vi "Draw Line.vi"(6 "Colour":u32(colorbox), 9 "Point 2":T1, 10 "Point 1":T1, 11 "Pixels":refnum<data-value>) -> (3 "Pixels (dup)":refnum<data-value>)   [LabVIEW 2020, in "Raster.lvlib"]
uses:
  Raster.lvlib
  Point 2D.ctl
  <vilib>/Utility/High Resolution Relative Seconds.vi
  Utility/Utility.lvlib
panel:
  out "Processing Time [s]":dbl format="%.1p"
  out "Iteration":i32
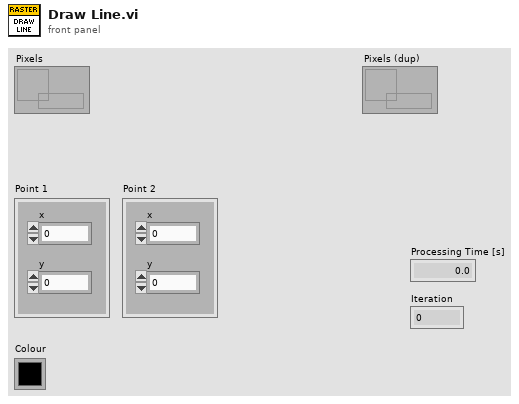
[diagram p1: front panel]
types:
  T1 = typedef "Raster.lvlib/Point 2D.ctl" = cluster{"x":i32, "y":i32}
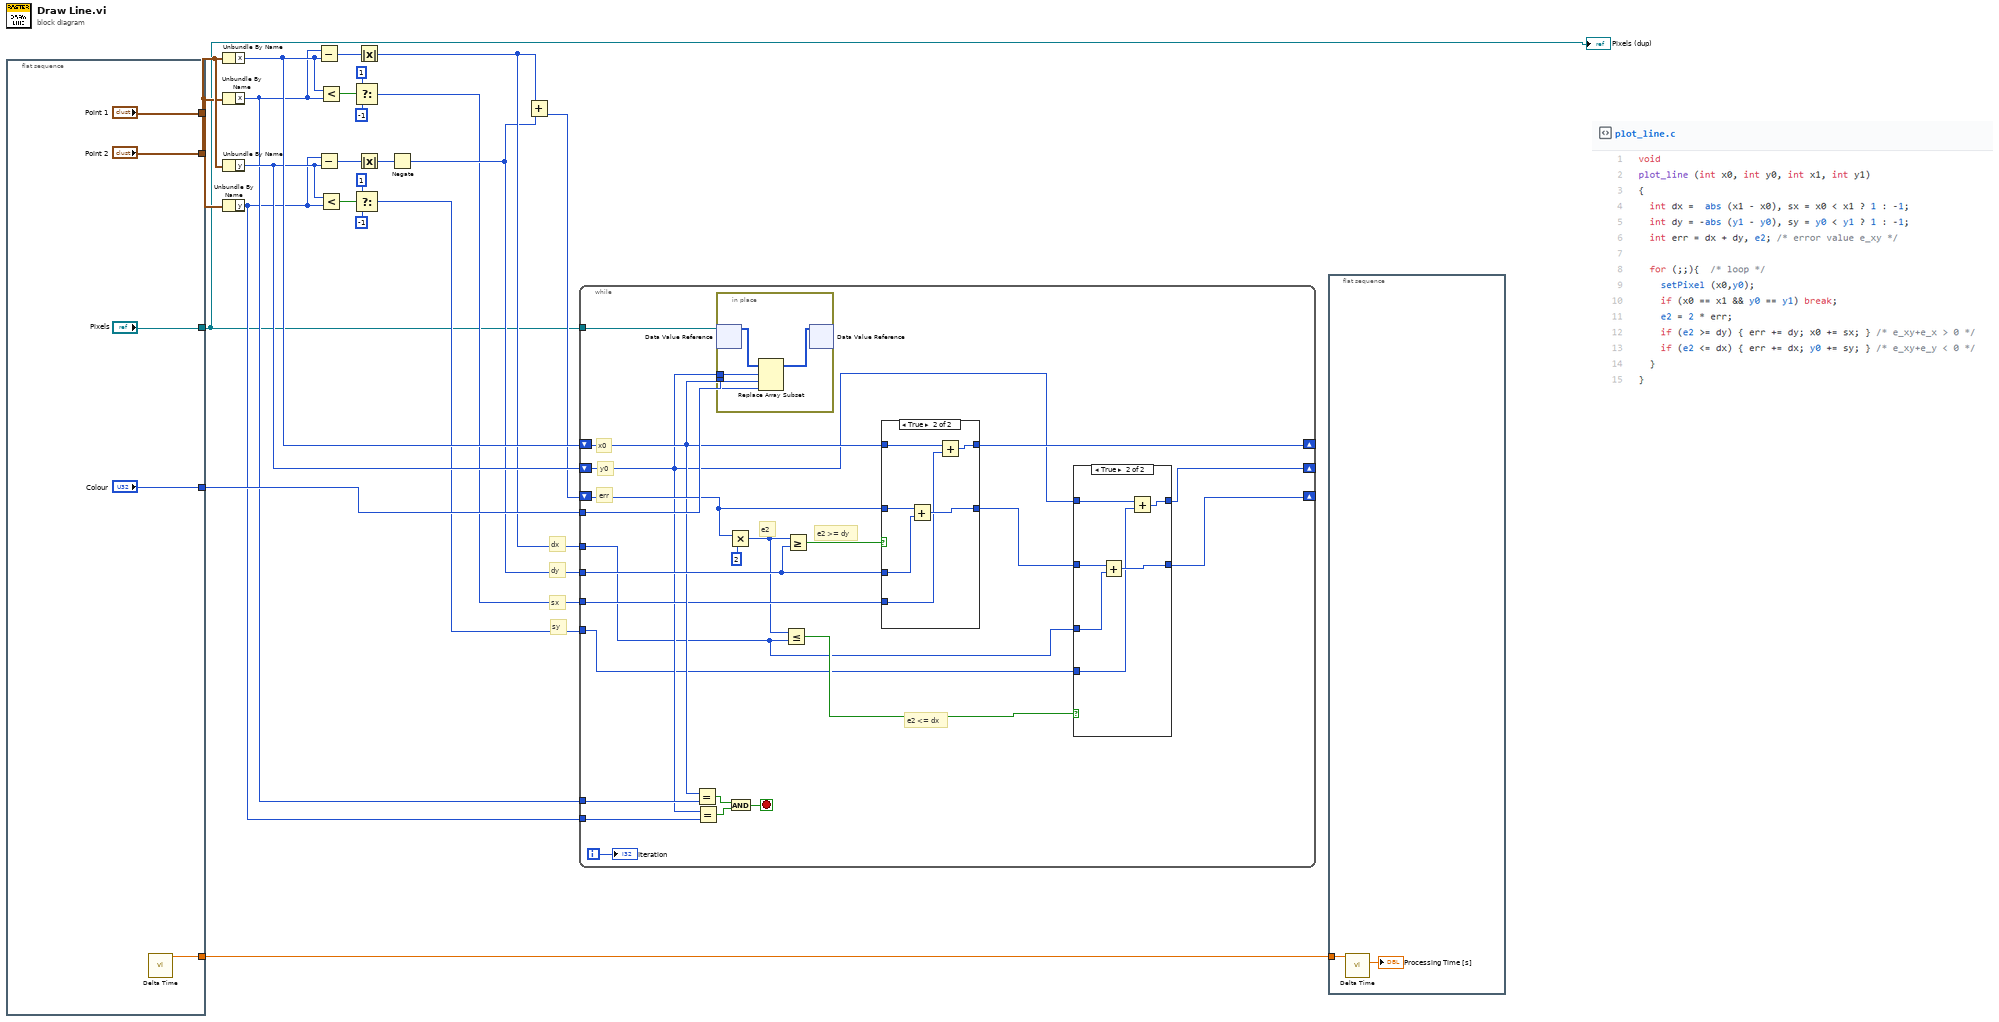
[diagram p0: block diagram]
diagram:
  # "sy"
  # "sx"
  # "dy"
  # "dx"
  n1 = flat-sequence {
    tunnel: ["Point 1"] -> w15
    tunnel: ["Point 2"] -> w14
    tunnel: ["Pixels"] -> w1
    tunnel: ["Colour"] -> w10
    tunnel: [w24] -> w2
    frame #0 {
      n2 = call "Delta Time.vi"() -> ("Relative Seconds Out"=w24:dbl)  [unwired: 10 in, 1 out]
    }
  }
  n3 = Unbundle By Name(w15) -> ("x"=w12:i32)
  n4 = Unbundle By Name(w14) -> ("x"=w9:i32)
  n5 = Unbundle By Name(w15) -> ("y"=w11:i32)
  n6 = Unbundle By Name(w14) -> ("y"=w8:i32)
  n7 = Subtract(x=w9, y=w12) -> (x-y=w23:i32)
  n8 = Subtract(x=w8, y=w11) -> (x-y=w16:i32)
  n9 = Less?(x=w12, y=w9) -> (x < y?=w22:bool)
  n10 = Less?(x=w11, y=w8) -> (x < y?=w17:bool)
  n11 = Select(t=1 ("x-y"), s=w22, f=-1 ("x-y")) -> (s? t:f=w4:i32)
  n12 = Select(t=1 ("x-y"), s=w17, f=-1 ("x-y")) -> (s? t:f=w3:i32)
  n13 = Absolute Value(x=w23) -> (abs(x)=w6:i32)
  n14 = Absolute Value(x=w16) -> (abs(x)=w13:i32)
  n15 = Negate(x=w13) -> (-x=w5:i32)
  n16 = Add(x=w6, y=w5) -> (x+y=w7:i32)
  n17 = while {
    shift-right: [w39] -> _
    shift-left: w12 -> [w41]
    shift-right: [w34] -> _
    shift-left: w11 -> [w35]
    tunnel: w10 -> [w51]
    tunnel: w9 -> [w50]
    tunnel: w8 -> [w49]
    shift-right: [w32] -> _
    shift-left: w7 -> [w43]
    tunnel: w6 -> [w33]
    tunnel: w5 -> [w42]
    tunnel: w4 -> [w40]
    tunnel: w3 -> [w31]
    tunnel: w1 -> [w29]
    i -> [w30]
    stop <- w46 stop-if-true
    # "e2 <= dx"
    # "e2 >= dy"
    # "e2"
    # "err"
    # "y0"
    # "x0"
    n18 = Equal?(x=w41, y=w50) -> (x = y?=w48:bool)
    n19 = Equal?(x=w35, y=w49) -> (x = y?=w47:bool)
    n20 = in-place {
      in-place-border: w51 -> [w56]
      in-place-border: w41 -> [w55]
      in-place-border: w35 -> [w54]
      n21 = in-place-dvr #1(w29) -> (w53:u32[][])  [unwired: 1 out]
      n22 = Replace Array Subset(array=w53, new element=w56, index (row)=w54, index (col)=w55) -> (w52:u32[][])
      n23 = in-place-dvr #1(w52) -> ()  [unwired: 2 out]
    }
    n24 = Multiply(x=w43, y=2) -> (x*y=w38:i32)
    n25 = And(x=w48, y=w47) -> (x .and. y?=w46:bool)
    n26 = Less Or Equal?(x=w38, y=w33) -> (x <= y?=w37:bool)
    n27 = Greater Or Equal?(x=w38, y=w42) -> (x >= y?=w44:bool)
    n28 = case shown="True" w44 {
      tunnel: w43 -> [w57 w64]
      tunnel: w42 -> [_ w63]
      tunnel: [w57 w62] -> w36
      tunnel: w41 -> [w58 w61]
      tunnel: w40 -> [_ w60]
      tunnel: [w58 w59] -> w39
      frame False {
      }
      frame True {
        n29 = Add(x=w64, y=w63) -> (x+y=w62:i32)
        n30 = Add(x=w61, y=w60) -> (x+y=w59:i32)
      }
    }
    n31 = case shown="True" w37 {
      tunnel: w36 -> [w66 w72]
      tunnel: w33 -> [_ w71]
      tunnel: [w66 w70] -> w32
      tunnel: w35 -> [w65 w69]
      tunnel: w31 -> [_ w68]
      tunnel: [w65 w67] -> w34
      frame False {
      }
      frame True {
        n32 = Add(x=w72, y=w71) -> (x+y=w70:i32)
        n33 = Add(x=w69, y=w68) -> (x+y=w67:i32)
      }
    }
    "Iteration" <- w30
  }
  n34 = flat-sequence {
    tunnel: w2 -> [w74]
    frame #0 {
      n35 = call "Delta Time.vi"("Relative Seconds In"=w74) -> ("Delta Time [s]"=→"Processing Time [s]":dbl)  [unwired: 9 in, 1 out]
    }
  }
  "Pixels (dup)" <- w1
